vi "XML_Get_General_Settings_Error_Checking.vi"(6 "General Settings":T1={"Communication_Type"=0, "Modbus_Type"=0, "Read_Write_Loop_Period"=-1, "TCP Settings"={"TCP_Settings_Port"=0, "TCP_Settings_IP_Timeout"=0, "TCP_Settings_IP_Slave_Address"=""}, "Serial Settings"={"Serial_Settings_Flow_Control"=0, "Serial_Settings_Baud_Rate"=0, "Serial_Settings_Parity"=0, "Serial_Settings_Resource_Name"="", "Serial_Settings_Serial_Type"=0, "Serial_Settings_Unit_ID"=0}} {"Communication_Type" items=["TCP", "Serial"]; "Modbus_Type" items=["Master", "Slave"]; "Serial Settings"."Serial_Settings_Flow_Control" items=["None", "XONXOFF", "RTSCTS", "XONXOFFANDRTSCTS", "DTRDSR", "XONXOFFANDDTRDSR"]; "Serial Settings"."Serial_Settings_Parity" items=["None", "Odd", "Even"]; "Serial Settings"."Serial_Settings_Serial_Type" items=["RTU", "ASCII"]}, 8 "error in (no error)":errorcluster, 9 "Read_Write_Loop_Period":i64, 10 "Modbus_Type":i32(ring) items=["Undefined", "Master", "Slave"], 11 "Communication_Type":i32(ring) items=["Undefined", "TCP", "Serial"]) -> (0 "error out":errorcluster, 3 "General Settings":T1={"Communication_Type"=0, "Modbus_Type"=0, "Read_Write_Loop_Period"=-1, "TCP Settings"={"TCP_Settings_Port"=0, "TCP_Settings_IP_Timeout"=0, "TCP_Settings_IP_Slave_Address"=""}, "Serial Settings"={"Serial_Settings_Flow_Control"=0, "Serial_Settings_Baud_Rate"=0, "Serial_Settings_Parity"=0, "Serial_Settings_Resource_Name"="", "Serial_Settings_Serial_Type"=0, "Serial_Settings_Unit_ID"=0}} {"Communication_Type" items=["TCP", "Serial"]; "Modbus_Type" items=["Master", "Slave"]; "Serial Settings"."Serial_Settings_Flow_Control" items=["None", "XONXOFF", "RTSCTS", "XONXOFFANDRTSCTS", "DTRDSR", "XONXOFFANDDTRDSR"]; "Serial Settings"."Serial_Settings_Parity" items=["None", "Odd", "Even"]; "Serial Settings"."Serial_Settings_Serial_Type" items=["RTU", "ASCII"]})   [LabVIEW 2014, in "XML_Deserializer.lvlib"]
uses:
  XML_Deserializer.lvlib
  Controls/Modbus_General_Settings.ctl
  Controls/Modbus_Communication_Type.ctl
  Controls/Modbus_Type.ctl
  Controls/Modbus_Serial_Settings_Flow_Control.ctl
  Controls/Modbus_Serial_Settings_Parity.ctl
  Controls/Modbus_Serial_Settings_Serial_Type.ctl
  Shared/Modbus Shared.lvlib
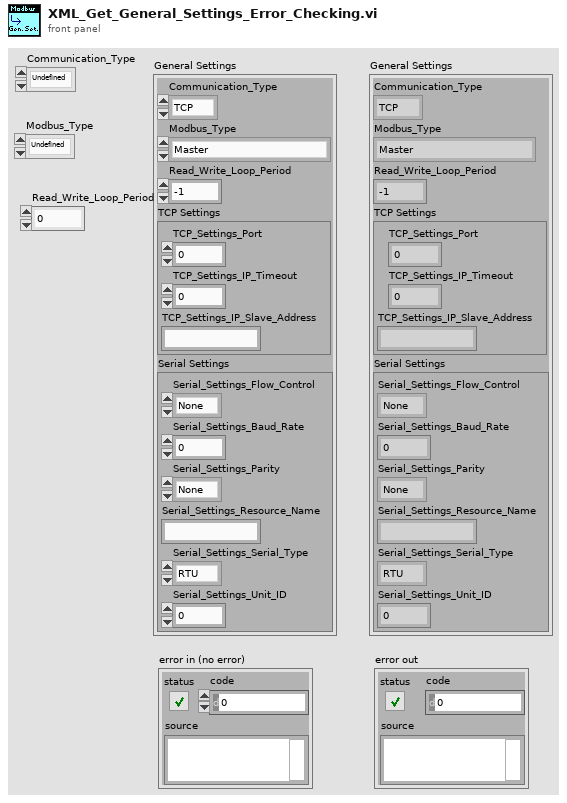
[diagram p1: front panel]
types:
  T1 = typedef "Modbus Shared.lvlib/Modbus_General_Settings.ctl" = cluster{"Communication_Type":T2, "Modbus_Type":T3, "Read_Write_Loop_Period":i64, "TCP Settings":cluster{"TCP_Settings_Port":u16, "TCP_Settings_IP_Timeout":u32, "TCP_Settings_IP_Slave_Address":string}, "Serial Settings":cluster{"Serial_Settings_Flow_Control":T4, "Serial_Settings_Baud_Rate":u32, "Serial_Settings_Parity":T5, "Serial_Settings_Resource_Name":string, "Serial_Settings_Serial_Type":T6, "Serial_Settings_Unit_ID":u8}}
  T2 = typedef "Modbus Shared.lvlib/Modbus_Communication_Type.ctl" = i32
  T3 = typedef "Modbus Shared.lvlib/Modbus_Type.ctl" = i32
  T4 = typedef "Modbus Shared.lvlib/Modbus_Serial_Settings_Flow_Control.ctl" = i32
  T5 = typedef "Modbus Shared.lvlib/Modbus_Serial_Settings_Parity.ctl" = i32
  T6 = typedef "Modbus Shared.lvlib/Modbus_Serial_Settings_Serial_Type.ctl" = i32
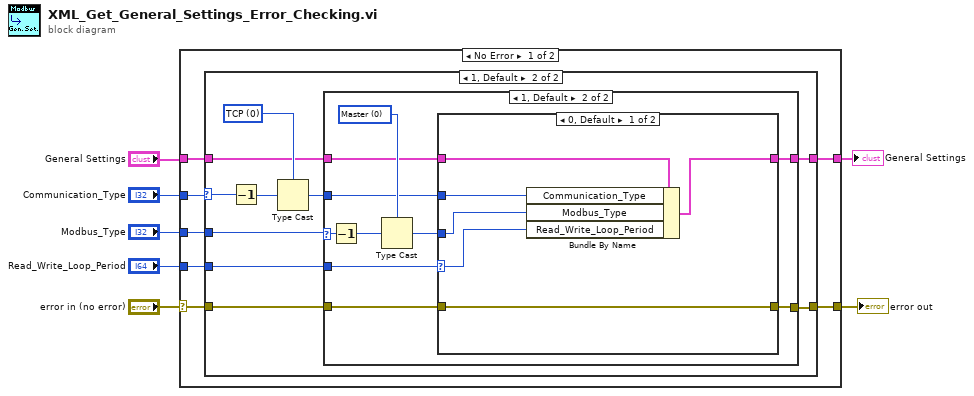
[diagram p0: block diagram]
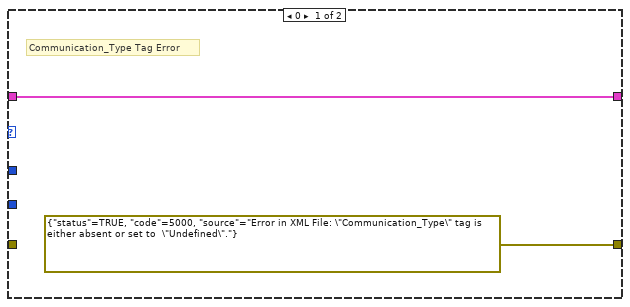
[diagram p2: hidden frame]
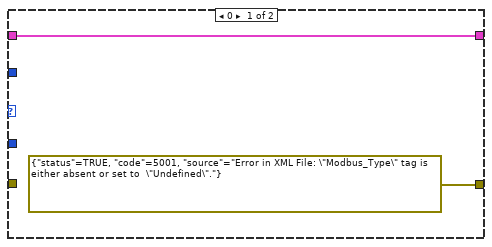
[diagram p3: hidden frame]
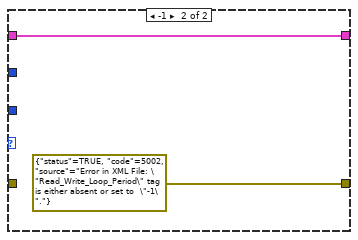
[diagram p4: hidden frame]
diagram:
  n1 = case shown="No Error" "error in (no error)" {
    selector: "error in (no error)" -> [w13 w48]
    tunnel: [w11 w48] -> w5
    tunnel: "General Settings" -> [w12 w47]
    tunnel: [w10 w47] -> w7
    tunnel: "Communication_Type" -> [w14 _]
    tunnel: "Modbus_Type" -> [w9 _]
    tunnel: "Read_Write_Loop_Period" -> [w8 _]
    frame No Error {
      n2 = case shown="1, Default" w14 {
        selector: w14 -> [_ w26]
        tunnel: w13 -> [_ w22]
        tunnel: w12 -> [w15 w20]
        tunnel: [errorcluster {"status"=TRUE, "code"=5000, "source"="Error in XML File: \"Communication_Type\" tag is either absent or set to  \"Undefined\"."} ("error out") w21] -> w11
        tunnel: [w15 w17] -> w10
        tunnel: w9 -> [_ w23]
        tunnel: w8 -> [_ w18]
        frame 0 {
          # "Communication_Type Tag Error"
        }
        frame 1, Default {
          w24 = T2 0 items=["TCP", "Serial"] ("Communication_Type 2")
          n3 = Decrement(x=w26) -> (x-1=w25:i32)
          n4 = Type Cast(type=w24, x=w25) -> (*(type *) &x=w19:T2)
          n5 = case shown="1, Default" w23 {
            selector: w23 -> [_ w38]
            tunnel: w22 -> [_ w30]
            tunnel: [errorcluster {"status"=TRUE, "code"=5001, "source"="Error in XML File: \"Modbus_Type\" tag is either absent or set to  \"Undefined\"."} ("error out") w29] -> w21
            tunnel: w20 -> [w27 w34]
            tunnel: w19 -> [_ w33]
            tunnel: w18 -> [_ w35]
            tunnel: [w27 w31] -> w17
            frame 0 {
            }
            frame 1, Default {
              w37 = T3 0 items=["Master", "Slave"] ("Modbus_Type 2")
              n6 = Decrement(x=w38) -> (x-1=w36:i32)
              n7 = Type Cast(type=w37, x=w36) -> (*(type *) &x=w32:T3)
              n8 = case shown="0, Default" w35 {
                selector: w35 -> [w41 _]
                tunnel: w34 -> [w44 w46]
                tunnel: w33 -> [w43 _]
                tunnel: w32 -> [w42 _]
                tunnel: [w40 w46] -> w31
                tunnel: w30 -> [w39 _]
                tunnel: [w39 errorcluster {"status"=TRUE, "code"=5002, "source"="Error in XML File: \"Read_Write_Loop_Period\" tag is either absent or set to  \"-1\"."} ("error out")] -> w29
                frame 0, Default {
                  n9 = Bundle By Name(cluster=w44, "Communication_Type"=w43, "Modbus_Type"=w42, "Read_Write_Loop_Period"=w41) -> (w40:T1)
                }
                frame -1 {
                }
              }
            }
          }
        }
      }
    }
    frame Error {
    }
  }
  "General Settings" <- w7
  "error out" <- w5
